vi "Open Hardware.vi"(8 "error in (no error)":errorcluster, 11 "Inst.Xeryon-Rotator in":refnum<class "Inst.Xeryon-Rotator.lvclass">) -> (0 "error out":errorcluster, 3 "Inst.Xeryon-Rotator out":refnum<class "Inst.Xeryon-Rotator.lvclass">)   [LabVIEW 2019, in "Inst.Xeryon-Rotator.lvclass"]
uses:
  Inst.Xeryon-Rotator.lvclass
  C:/Program Files/National Instruments/LabVIEW 2019/user.lib/LevyLab/Instrument Framework/Instrument/Instrument.lvclass
  <userlib>/LevyLab/Instrument Framework/Instrument/Instrument.lvclass/Instrument.ctl
  Controller.LV/Controller.LV.lvclass
  Inst.Xeryon-Rotator.lvclass/Inst.Xeryon-Rotator.ctl
  <userlib>/LevyLab/Instrument Framework/Instrument Types/Cryostat/Instrument.Cryostat.lvclass
  <userlib>/LevyLab/Instrument Framework/Instrument/Instrument.lvclass
  C:/Program Files/National Instruments/LabVIEW 2019/user.lib/LevyLab/Instrument Framework/Instrument Types/Cryostat/Instrument.Cryostat.lvclass
  C:/Program Files/National Instruments/LabVIEW 2019/vi.lib/JKI/JKI SMO/SMO/SMO.lvclass
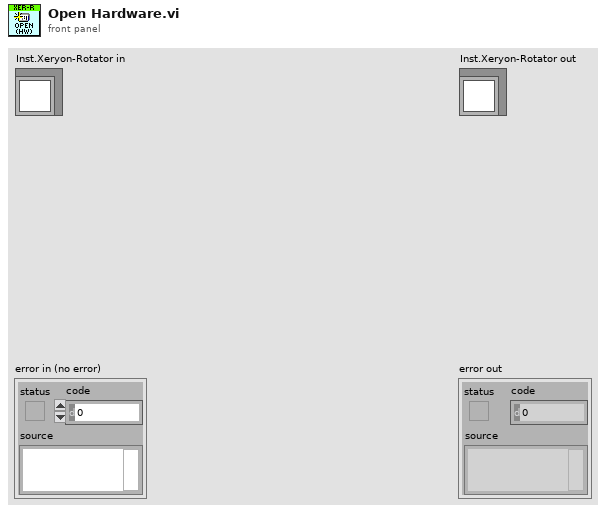
[diagram p1: front panel]
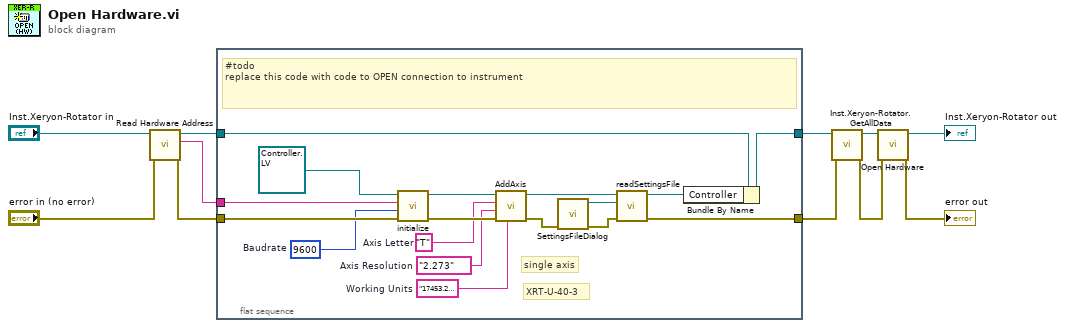
[diagram p0: block diagram]
diagram:
  n1 = call <userlib>:"Read Hardware Address.vi"("error in (no error)"="error in (no error)", "Instrument in"="Inst.Xeryon-Rotator in") -> ("error out"=w11:errorcluster, "Address"=w10:string, "Instrument out"=w9:refnum<class "Inst.Xeryon-Rotator.lvclass">)  [unwired: 7 in]
  n2 = flat-sequence {
    tunnel: w9 -> [w28]
    tunnel: [w27] -> w4
    tunnel: w11 -> [w24]
    tunnel: [w16] -> w2
    tunnel: w10 -> [w22]
    frame #0 {
      w21 = "17453.292519943294"  # Working Units
      w19 = "2.273"  # Axis Resolution
      w18 = "T"  # Axis Letter
      w20 = u32 9600  # Baudrate
      # "single axis"
      # "XRT-U-40-3"
      # "#todo\nreplace this code with code to OPEN connection to instrument"
      n3 = call-dynamic "initialize.vi"("error in (no error)"=w24, "Baudrate"=w20, "COM Port"=w22, "Controller in"=refnum<class "Controller.LV.lvclass"> refnum ("Controller.LV.lvclass")) -> ("error out"=w23:errorcluster, "Controller out"=w25:refnum<class "Controller.LV.lvclass">)  [unwired: 6 in]
      n4 = call-dynamic "AddAxis.vi"("Units"=w21, "error in (no error)"=w23, "Encoder Resolution"=w19, "Axis Letter"=w18, "Controller in"=w25) -> ("error out"=w13:errorcluster, "Controller out"=w26:refnum<class "Controller.LV.lvclass">)  [unwired: 5 in]
      n5 = call "SettingsFileDialog.vi"("error in (no error)"=w13) -> ("error out"=w12:errorcluster, "selected path"=w14:path)  [unwired: 9 in]
      n6 = call-dynamic "readSettingsFile.vi"("error in (no error)"=w12, "file (use dialog)"=w14, "Controller in"=w26) -> ("error out"=w16:errorcluster, "Controller out"=w17:refnum<class "Controller.LV.lvclass">)  [unwired: 7 in]
      n7 = Bundle By Name(cluster=w28, "Controller"=w17) -> (w27:refnum<class "Inst.Xeryon-Rotator.lvclass">)
    }
  }
  n8 = call "Inst.Xeryon-Rotator.GetAllData.vi"("error in (no error)"=w2, "Inst.Xeryon-Rotator in"=w4) -> ("error out"=w1:errorcluster, "Inst.Xeryon-Rotator out"=w3:refnum<class "Inst.Xeryon-Rotator.lvclass">)  [unwired: 7 in, 1 out]
  n9 = call-parent "Open Hardware.vi"("error in (no error)"=w1, "Instrument in"=w3) -> ("error out"=→"error out":errorcluster, "Instrument out"=→"Inst.Xeryon-Rotator out":refnum<class "Inst.Xeryon-Rotator.lvclass">)  [unwired: 8 in]
